vi "map.vi"() -> ()   [LabVIEW 2019]
panel:
  out "거리":dbl[](array[numeric])
  out "수정된 로봇의 회전각":dbl[](array[numeric])=[-45.0, 90.0, -45.0]
  out "로봇의 회전각":dbl
  out "dot2dot degree":dbl=90.0
  in  "배열":dbl[][](array[numeric])=[[1.0, 1.0], [0.0, 2.0], [0.0, 3.0]]
  # "1. 행렬로 좌표값이 들어옴(행렬에 두개의 요소A,B / A(x1,y1)->B(x2,y2)순서라고 가정)\n2-1. 0도 \n     x1-x2=1, y1-y2=0"
  # "돌고->가고"
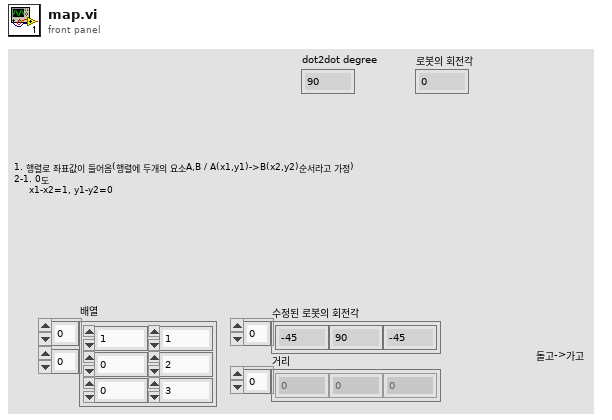
[diagram p1: front panel]
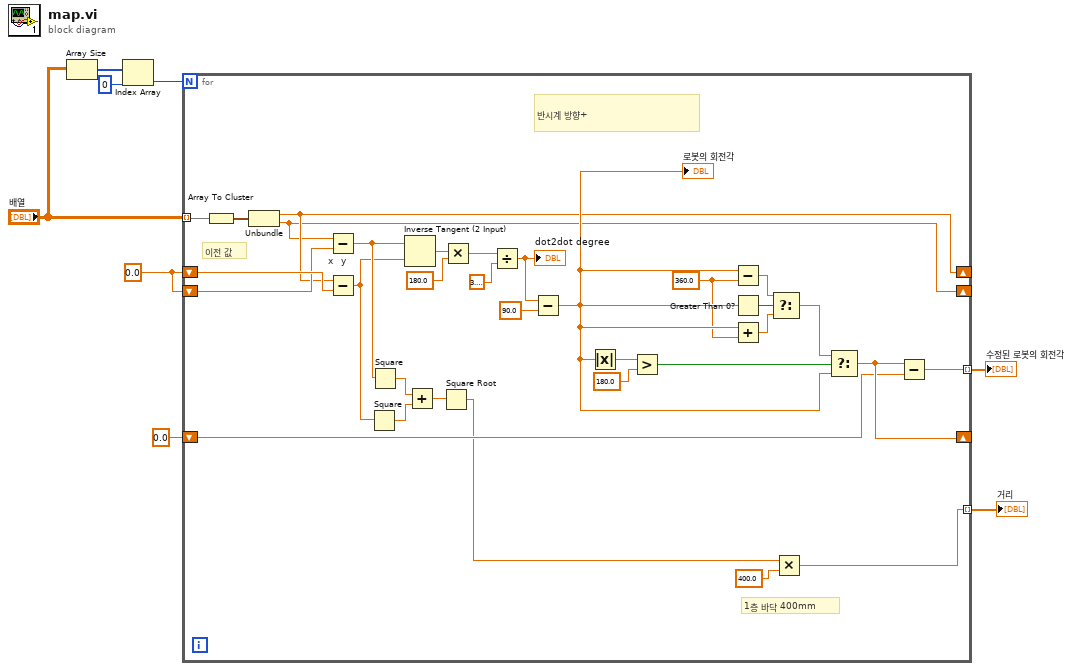
[diagram p0: block diagram]
diagram:
  w4 = 0.0 ("y")
  n1 = Array Size(array="배열") -> (size(s)=w7:i32[])
  n2 = Index Array(array=w7, index=0 ("인덱스")) -> (element=w5:i32)
  n3 = for {
    N: w5 -> [_]
    tunnel: "배열" -> [w40] mode=indexing
    shift-right: [w21] -> _
    shift-left: w4 -> [w23]
    shift-right: [w20] -> _
    shift-left: w4 -> [w22]
    shift-right: [w19] -> _
    shift-left: 0.0 -> [w18]
    tunnel: [w17] -> w2 mode=indexing
    tunnel: [w10] -> w1 mode=indexing
    w24 = 360.0 ("y")
    # "1층 바닥 400mm"
    # "이전 값"
    # "반시계 방향+"
    n4 = Array To Cluster(array=w40) -> (cluster=w39:cluster{"배열[0]":dbl, "배열[1]":dbl})
    n5 = Unbundle(w39) -> ("배열[0]"=w21:dbl, "배열[1]"=w20:dbl)
    n6 = Subtract "y"(x=w20, y=w22) -> (x-y=w13:dbl)
    n7 = Subtract "x"(x=w21, y=w23) -> (x-y=w12:dbl)
    n8 = Square(x=w12) -> (x^2=w14:dbl)
    n9 = Square(x=w13) -> (x^2=w15:dbl)
    n10 = Inverse Tangent (2 Input)(1:w12, 2:w13) -> (0:w38:dbl)
    n11 = Add(x=w15, y=w14) -> (x+y=w16:dbl)
    n12 = Square Root(x=w16) -> (sqrt(x)=w9:dbl)
    n13 = Multiply(x=w38, y=180.0) -> (x*y=w36:dbl)
    n14 = Divide(x=w36, y=3.141592653589793) -> (x/y=w33:dbl)
    "dot2dot degree" <- w33
    n15 = Subtract(x=w33, y=90.0) -> (x-y=w25:dbl)
    "로봇의 회전각" <- w25
    n16 = Absolute Value(x=w25) -> (abs(x)=w32:dbl)
    n17 = Greater?(x=w32, y=180.0) -> (0:w30:bool)
    n18 = Subtract(x=w25, y=w24) -> (x-y=w27:dbl)
    n19 = Greater Than 0?(x=w25) -> (x > 0?=w29:bool)
    n20 = Add(x=w25, y=w24) -> (x+y=w26:dbl)
    n21 = Select(t=w27, s=w29, f=w26) -> (s? t:f=w28:dbl)
    n22 = Multiply(x=w9, y=400.0) -> (x*y=w10:dbl)
    n23 = Select(t=w28, s=w30, f=w25) -> (s? t:f=w19:dbl)
    n24 = Subtract(x=w19, y=w18) -> (x-y=w17:dbl)
  }
  "수정된 로봇의 회전각" <- w2
  "거리" <- w1
